vi "get servo angles.vi"() -> ()   [LabVIEW 2022 SP3]
panel:
  out "Numeric":i32
  out "Numeric 4":i32
  out "Numeric 3":i32
  out "Numeric 2":i32
  in  "Slide":i32(slide) scale=0.0..10.0
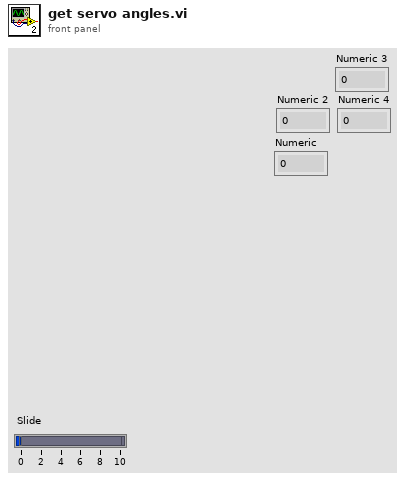
[diagram p1: front panel]
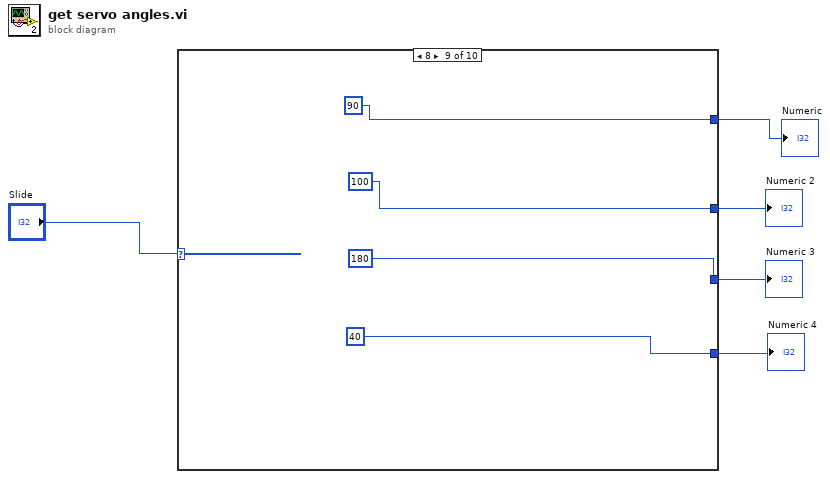
[diagram p0: block diagram]
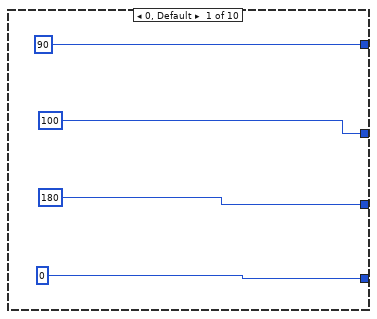
[diagram p2: hidden frame]
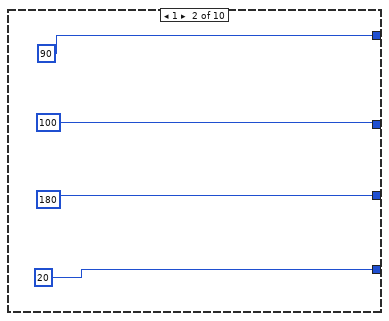
[diagram p3: hidden frame]
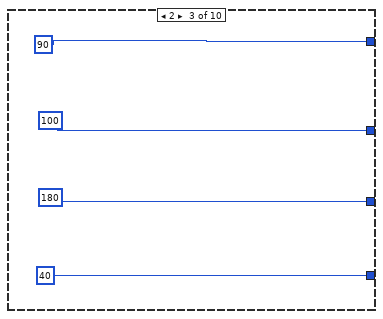
[diagram p4: hidden frame]
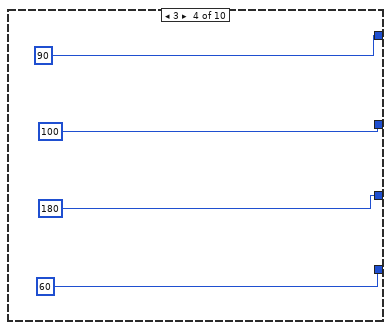
[diagram p5: hidden frame]
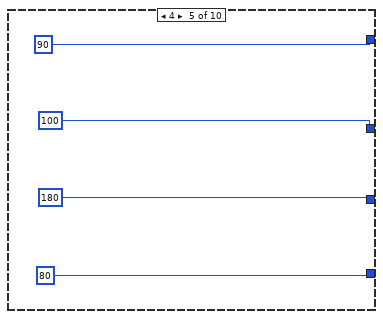
[diagram p6: hidden frame]
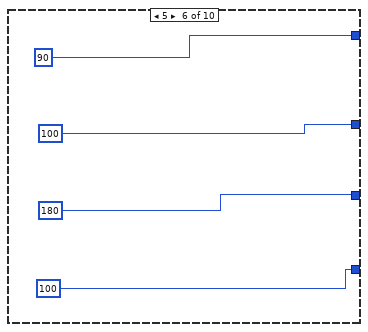
[diagram p7: hidden frame]
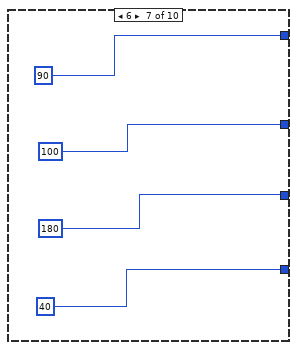
[diagram p8: hidden frame]
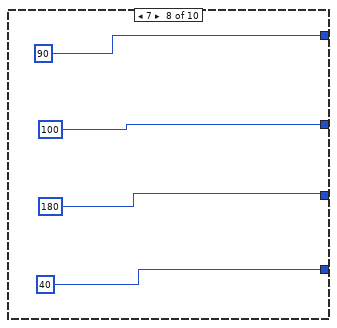
[diagram p9: hidden frame]
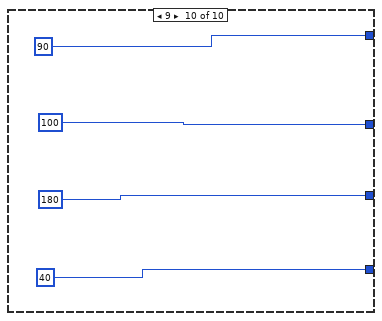
[diagram p10: hidden frame]
diagram:
  n1 = case shown="8" "Slide" {
    tunnel: [100 100 100 100 100 100 100 100 100 100] -> w4
    tunnel: [180 180 180 180 180 180 180 180 180 180] -> w3
    tunnel: [0 20 40 60 80 100 40 40 40 40] -> w2
    tunnel: [90 90 90 90 90 90 90 90 90 90] -> w1
    frame 0, Default {
    }
    frame 1 {
    }
    frame 2 {
    }
    frame 3 {
    }
    frame 4 {
    }
    frame 5 {
    }
    frame 6 {
    }
    frame 7 {
    }
    frame 8 {
    }
    frame 9 {
    }
  }
  "Numeric 2" <- w4
  "Numeric 3" <- w3
  "Numeric 4" <- w2
  "Numeric" <- w1
